vi "SpinCoaterArray2String_v05.vi"(3 "Time Start":dbl[unit], 4 "Program Spin Coater\nSpeed (rpm)          Time (s)":dbl[][](array[numeric]), 5 "Time Spin":dbl[unit]) -> (0 "Prg Spin Coater small":dbl[][](array[numeric]), 1 "remote control String":string)   [LabVIEW 2020, in "SpinCoater.lvclass"]
uses:
  <instrlib>/Classes/SpinCoater/SpinCoater.lvclass
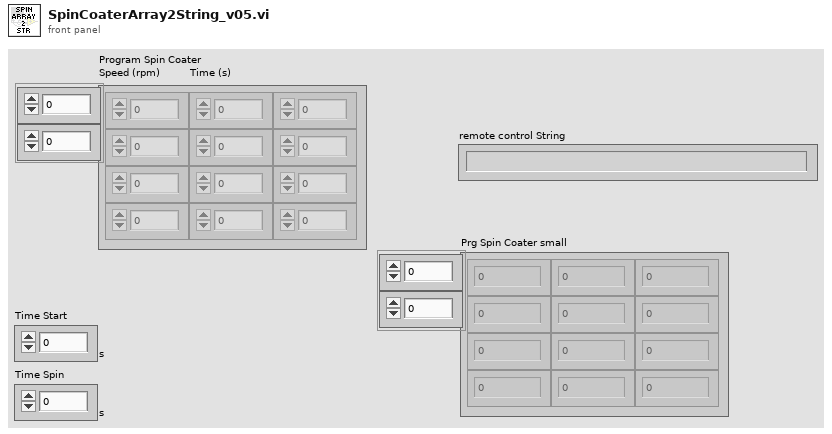
[diagram p1: front panel]
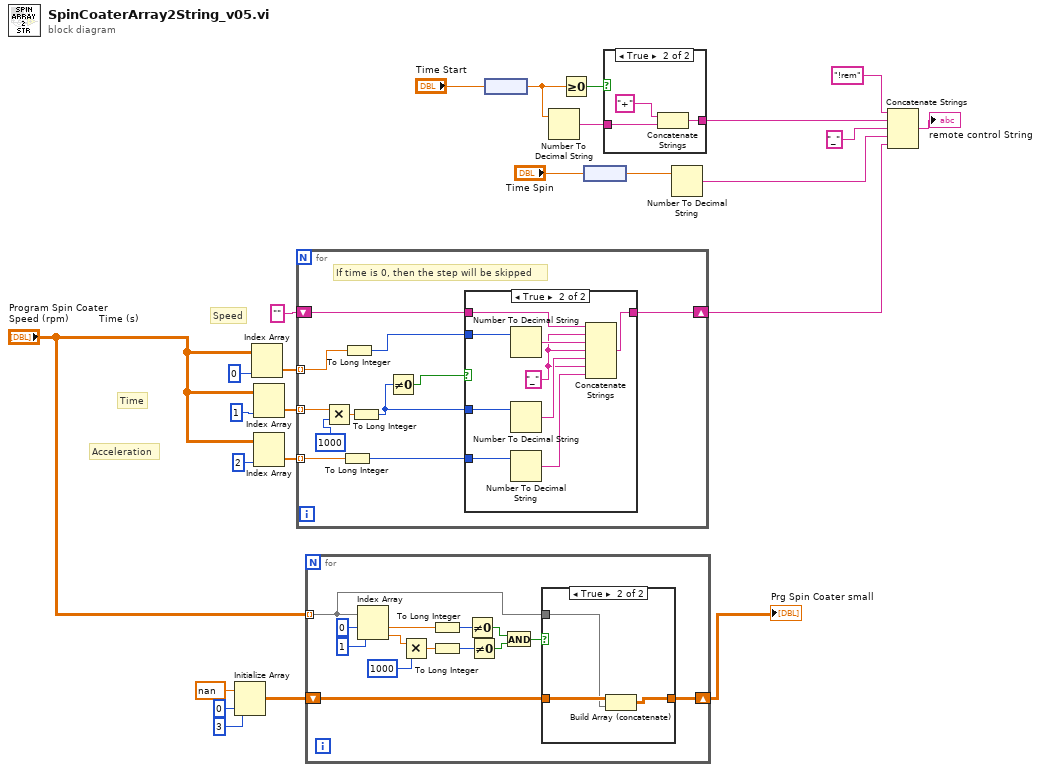
[diagram p0: block diagram]
diagram:
  # "Acceleration"
  # "Time"
  # "Speed"
  n1 = Initialize Array(nan ("element"), 0 ("dimension size"), 3 ("dimension size")) -> (w7:dbl[][])
  n2 = Index Array(array="Program Spin Coater\nSpeed (rpm)          Time (s)", index (col)=0 ("disabled index (col)")) -> (element=w23:dbl[])  [unwired: 1 in]
  n3 = Index Array(array="Program Spin Coater\nSpeed (rpm)          Time (s)", index (col)=1 ("disabled index (col)")) -> (element=w22:dbl[])  [unwired: 1 in]
  n4 = Index Array(array="Program Spin Coater\nSpeed (rpm)          Time (s)", index (col)=2 ("disabled index (col)")) -> (element=w12:dbl[])  [unwired: 1 in]
  n5 = for {
    tunnel: w23 -> [w36] mode=indexing
    tunnel: w22 -> [w29] mode=indexing
    shift-right: [w33] -> w1
    shift-left: "" ("string") -> [w34]
    tunnel: w12 -> [w32] mode=indexing
    # "If time is 0, then the step will be skipped"
    n6 = Multiply(x=w29, y=1000) -> (x*y=w30:dbl)
    n7 = To Long Integer(number=w32) -> (32bit integer=w31:i32)
    n8 = To Long Integer(number=w36) -> (32bit integer=w35:i32)
    n9 = To Long Integer(number=w30) -> (32bit integer=w27:i32)
    n10 = Not Equal To 0?(x=w27) -> (x != 0?=w26:bool)
    n11 = case shown="True" w26 {
      tunnel: w35 -> [_ w46]
      tunnel: w27 -> [_ w45]
      tunnel: w34 -> [w37 w42]
      tunnel: [w37 w41] -> w33
      tunnel: w31 -> [_ w40]
      frame False {
      }
      frame True {
        w39 = "_" ("string")
        n12 = Number To Decimal String(number=w46) -> (decimal integer string=w44:string)  [unwired: 1 in]
        n13 = Number To Decimal String(number=w45) -> (decimal integer string=w43:string)  [unwired: 1 in]
        n14 = Number To Decimal String(number=w40) -> (decimal integer string=w38:string)  [unwired: 1 in]
        n15 = Concatenate Strings(w42, w39, w44, w39, w43, w39, w38) -> (w41:string)
      }
    }
  }
  n16 = for {
    tunnel: "Program Spin Coater\nSpeed (rpm)          Time (s)" -> [w52] mode=indexing
    shift-right: [w50] -> w6
    shift-left: w7 -> [w51]
    n17 = Index Array(array=w52, index #1=0 ("index"), index #2=1 ("index")) -> (element #1=w58:dbl, element #2=w48:dbl)
    n18 = Multiply(x=w48, y=1000) -> (x*y=w49:dbl)
    n19 = To Long Integer(number=w58) -> (32bit integer=w54:i32)
    n20 = To Long Integer(number=w49) -> (32bit integer=w55:i32)
    n21 = Not Equal To 0?(x=w54) -> (x != 0?=w57:bool)
    n22 = Not Equal To 0?(x=w55) -> (x != 0?=w56:bool)
    n23 = And(x=w57, y=w56) -> (x .and. y?=w53:bool)
    n24 = case shown="True" w53 {
      tunnel: w52 -> [_ w63]
      tunnel: w51 -> [w61 w64]
      tunnel: [w61 w62] -> w50
      frame False {
      }
      frame True {
        n25 = Build Array (concatenate)(w64, w63) -> (w62:dbl[][])
      }
    }
  }
  "Prg Spin Coater small" <- w6
  n26 = node("Time Start") -> (w17:dbl)
  n27 = Number To Decimal String(number=w17) -> (decimal integer string=w16:string)  [unwired: 1 in]
  n28 = Greater Or Equal To 0?(x=w17) -> (x >= 0?=w18:bool)
  n29 = node("Time Spin") -> (w4:dbl)
  n30 = case shown="True" w18 {
    tunnel: w16 -> [w65 w67]
    tunnel: [w65 w66] -> w15
    frame False {
    }
    frame True {
      n31 = Concatenate Strings("+", w67) -> (w66:string)
    }
  }
  n32 = Number To Decimal String(number=w4) -> (decimal integer string=w2:string)  [unwired: 1 in]
  n33 = Concatenate Strings("!rem" ("string"), w15, "_" ("string"), w2, w1) -> (→"remote control String":string)
